vi "GetDataCollectorChannel.vi"(8 "error in (no error)":errorcluster, 11 "reference in":refnum<class "DAQ_Base.lvclass">) -> (0 "error out":errorcluster, 2 "DataCollectorChannel":T1, 3 "reference out":refnum<class "DAQ_Base.lvclass">)   [LabVIEW 2020]
uses:
  DAQ_Base.lvclass
  protected/DataCollector.ctl
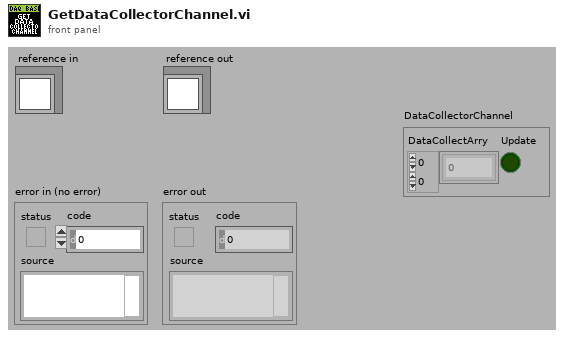
[diagram p1: front panel]
types:
  T1 = typedef "DAQ_Base.lvclass/DataCollector.ctl" = cluster{"DataCollectArry":dbl[][], "Update":bool}
  T2 = typedef "DAQ_Base.lvclass/ObjectAttributesRef.ctl" = refnum<data-value>
  T3 = typedef "DAQ_Base.lvclass/ObjectAttributes.ctl" = cluster{"MyAttribute":dbl, "RootPath":path, "DAQSettings":T4, "CollectorChannelEnable":bool[], "CollectDataQueue":refnum<queue>, "ArryDataCollectorChannel":T1[]}
  T4 = typedef "DAQ_Base.lvclass/DAQSettings.ctl" = cluster{"SampleSettings":T5, "AI_ChannelSettings":T6, "AO_ChannelSettings":T7, "Cnt_ChannelSettings":T8}
  T5 = typedef "DAQ_Base.lvclass/SampleSettings.ctl" = cluster{"samples per channel":i32, "SampleRate":dbl, "TansMaxLength":dbl, "ReadTimeOut":dbl, "时钟源":tag}
  T6 = typedef "DAQ_Base.lvclass/AI_ChannelSettings.ctl" = cluster{"AI_SettingsArry":cluster{"DeviceName":tag, "physical channels":tag, "AssignName":string, "输入信号类型":enum16{"默认", "RSE", "NRSE", "差分", "伪差分"}, "Max_value":dbl, "Min_value":dbl, "单位":enum16{"安培", "伏特", "来自自定义换算"}, "shunt resistor location":i32, "external shunt resistor value":dbl}[]}
  T7 = typedef "DAQ_Base.lvclass/AO_ChannelSettings.ctl" = cluster{"布尔":bool}
  T8 = typedef "DAQ_Base.lvclass/Cnt_ChannelSettings.ctl" = cluster{"Cnt_ChannelSettings":cluster{"类型":enum16{"Linear", "Rotate"}, "CounterNbr":tag, "AssignName":string, "单位":enum16{"Radians", "Degrees", "Meters", "Inches", "Ticks", "From Custom Scale"}, "decoding type":enum16{"X1", "X2", "X4", "双脉冲计数"}, "PPR_DistancePerPulse":dbl, "Initial Position ":dbl, "z index enable":bool, "z index phase":enum16{"A High B High", "A High B Low", "A Low B High", "A Low B Low"}, "source":tag}[]}
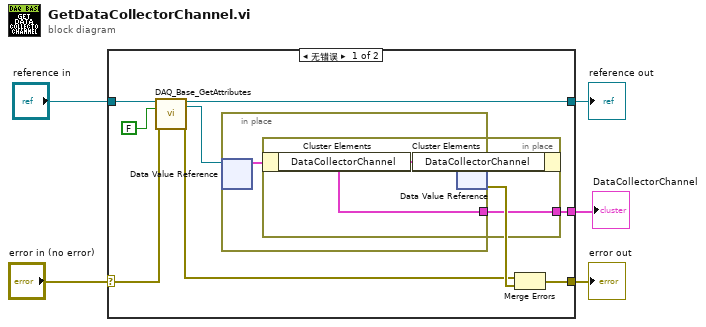
[diagram p0: block diagram]
diagram:
  n1 = case shown="无错误" "error in (no error)" {
    selector: "error in (no error)" -> [w14 w20]
    tunnel: [w8 w20] -> w4
    tunnel: [w13 w19] -> w2
    tunnel: "reference in" -> [w12 w19]
    tunnel: [w6 _] -> w1
    frame No Error {
      n2 = call "DAQ_Base_GetAttributes.vi"("reference in"=w12, "return data? (T)"=FALSE, "error in (no error)"=w14) -> ("reference out"=w13:refnum<class "DAQ_Base.lvclass">, "attributes ref"=w7:T2, "error out"=w9:errorcluster)  [unwired: 13 in, 1 out]
      n3 = in-place {
        in-place-border: [w15] -> w6
        n4 = in-place-dvr #1(w7) -> (w16:T3)  [unwired: 1 out]
        n5 = in-place {
          in-place-border: [w18] -> w15
          n6 = in-place-cluster #2(w16) -> ("DataCollectorChannel"=w18:T1)
          n7 = in-place-cluster #2("DataCollectorChannel"=w18) -> (w17:T3)
        }
        n8 = in-place-dvr #1(w17) -> (w10:errorcluster)  [unwired: 1 out]
      }
      n9 = Merge Errors(w9, w10) -> (w8:errorcluster)
    }
    frame Error {
    }
  }
  "error out" <- w4
  "reference out" <- w2
  "DataCollectorChannel" <- w1
